vi "power.vi"(8 "error in (no error)":errorcluster, 11 "AdvancedRemote in":refnum<class "AdvancedRemote.lvclass">) -> (0 "error out":errorcluster, 3 "AdvancedRemote out":refnum<class "AdvancedRemote.lvclass">)   [LabVIEW 2017, in "AdvancedRemote.lvclass"]
uses:
  AdvancedRemote.lvclass
  BasicRemote Class/BasicRemote.lvclass
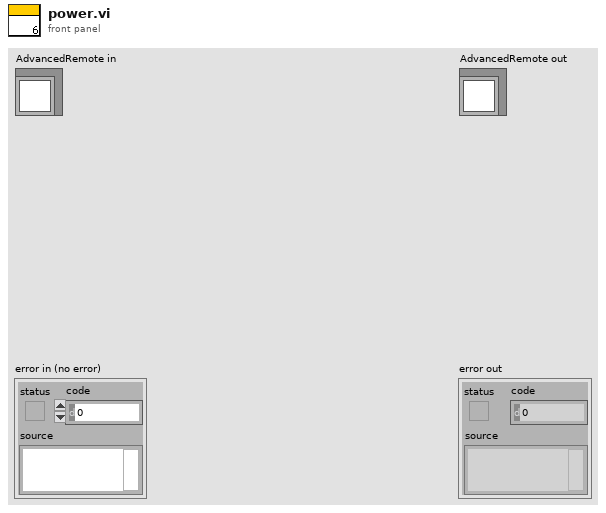
[diagram p1: front panel]
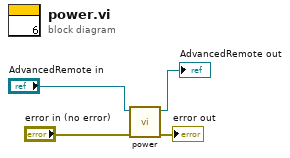
[diagram p0: block diagram]
diagram:
  n1 = call-parent "power.vi"("error in (no error)"="error in (no error)", "BasicRemote in"="AdvancedRemote in") -> ("error out"=→"error out":errorcluster, "BasicRemote out"=→"AdvancedRemote out":refnum<class "AdvancedRemote.lvclass">)  [unwired: 8 in]
